vi "Get All Properties.vi"(8 "error in (no error)":errorcluster, 11 "Service in":refnum<class "Service.lvclass">) -> (0 "error out":errorcluster, 2 "Properties":cluster{"Name":string, "Value":string}[](array[cluster]), 3 "Service out":refnum<class "Service.lvclass">)   [LabVIEW 2024, in "Ramses Framework.lvlib" / "Service.lvclass"]
uses:
  Service.lvclass
  Service.lvclass/Service.ctl
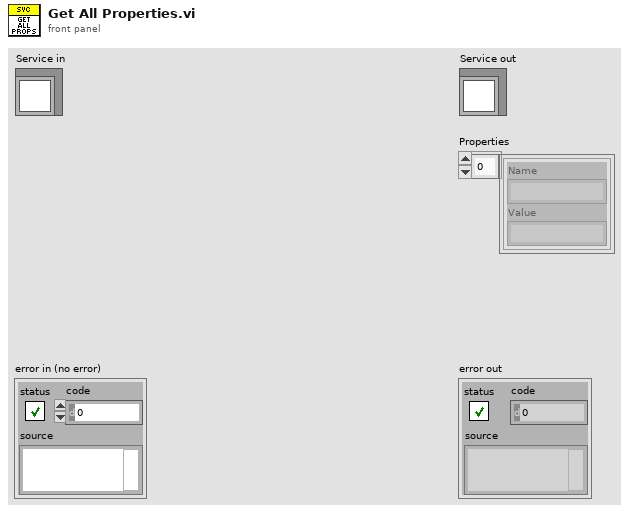
[diagram p1: front panel]
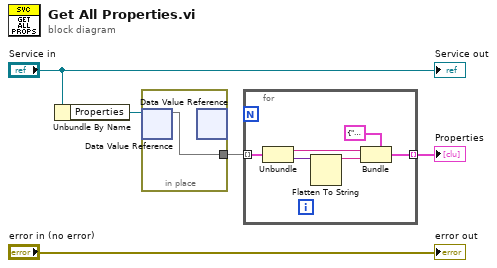
[diagram p0: block diagram]
diagram:
  n1 = Unbundle By Name("Service in") -> ("Properties"=w3:refnum<data-value>)
  n2 = in-place {
    in-place-border: [w6] -> w1
    n3 = in-place-dvr #1(w3) -> (w6:map{string, variant})  [unwired: 1 out]
    n4 = in-place-dvr #1() -> ()  [unwired: 1 in, 2 out]
  }
  n5 = for {
    tunnel: [w12] -> w2 mode=indexing
    tunnel: w1 -> [w9] mode=indexing
    n6 = Unbundle(w9) -> (w7:string, "Variant"=w8:variant)
    n7 = Flatten To String(anything=w8) -> (data string=w10:string)  [unwired: 3 in, 2 out]
    n8 = Bundle(cluster=cluster{"Name":string, "Value":string} {"Name"="", "Value"=""}, "Name"=w7, "Value"=w10) -> (w12:cluster{"Name":string, "Value":string})
  }
  "Properties" <- w2
  "error out" <- "error in (no error)"
  "Service out" <- "Service in"
